vi "Ticks to Rotations (Drive).vi"(11 "Drive Velocities (ticks)":T1) -> (3 "Drive Velocities (rotations)":T1)   [LabVIEW 2020]
uses:
  2023 Charged Up Robot Project/Framework/Robot Global Data.vi
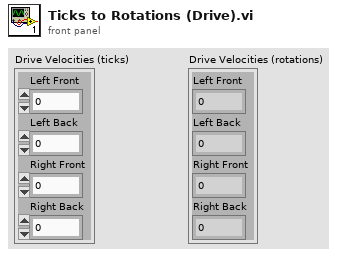
[diagram p1: front panel]
types:
  T1 = cluster{"Left Front":dbl, "Left Back":dbl, "Right Front":dbl, "Right Back":dbl}
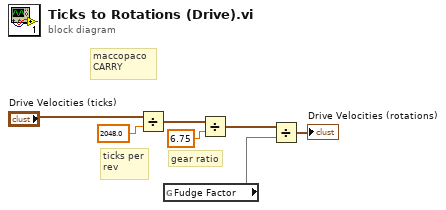
[diagram p0: block diagram]
diagram:
  # "ticks per\nrev"
  # "gear ratio"
  # "maccopaco\nCARRY"
  n1 = Divide(x="Drive Velocities (ticks)", y=2048.0) -> (x/y=w2:T1)
  n2 = global read "Robot Global Data.vi" "Fudge Factor"() -> (w4)
  n3 = Divide(x=w2, y=6.75) -> (x/y=w5:T1)
  n4 = Divide(x=w5, y=w4) -> (x/y=→"Drive Velocities (rotations)":T1)
